vi "Documentation.vi"   [LabVIEW 2019, in "Inst.RP100.lvlib" / "Inst.RP100.lvclass"]
uses:
  Inst.RP100.lvclass
  7f3c9b6f-0033-4804-bc48-630b6ca02c12.vi
  7f3c9b6f-0033-4804-bc48-630b6ca02c12.vi/dae691d2-a16d-43f7-880e-3d4c6070a6ed.vi
  7f3c9b6f-0033-4804-bc48-630b6ca02c12.vi/01ba8764-a54b-435f-b6e6-8e2e51a5d755.vi
  <userlib>/LevyLab/Instrument Framework/Instrument/API/Instrument.sendMessageToProcess (string).vi
  <vilib>/Utility/Data Type/Get Type Information.vi
  <vilib>/JDP Science/JSONtext/JSON text to Variant.vi
  <userlib>/LevyLab/Instrument Framework/Instrument/Instrument.lvclass
  <vilib>/JKI/JKI SMO/SMO/SMO.lvclass
  Typedefs/Inst.RP100.Commands--Enum.ctl
  Typedefs/Inst.RP100.getAll--Cluster.ctl
  Typedefs/Inst.RP100.Configuration--Cluster.ctl
  Inst UI.RP100/Inst UI.RP100.lvclass
  Inst UI.RP100/Inst UI.RP100.UI--Cluster.ctl
  <vilib>/JKI/JKI SMO/SMO.UI/SMO.UI.lvclass
  <userlib>/LevyLab/Instrument Framework/Instrument UI/Instrument UI.lvclass
  <vilib>/JDP Science/JSONtext/LVClass Serializer/JSONtext LVClass Serializer.lvclass
  <userlib>/LevyLab/RemoteControl/RemoteControl/RemoteControl.lvclass
  C:/Program Files (x86)/National Instruments/LabVIEW 2019/user.lib/LevyLab/Instrument Framework/Instrument Types/Strain/Instrument.Strain.lvclass
  C:/Program Files (x86)/National Instruments/LabVIEW 2019/user.lib/LevyLab/Instrument Framework/Instrument/Instrument.lvclass
  C:/Program Files (x86)/National Instruments/LabVIEW 2019/vi.lib/JKI/JKI SMO/SMO/SMO.lvclass
  C:/Program Files (x86)/National Instruments/LabVIEW 2019/user.lib/LevyLab/Instrument Framework/Instrument UI/Instrument UI.lvclass
  C:/Program Files (x86)/National Instruments/LabVIEW 2019/vi.lib/JKI/JKI SMO/SMO.UI/SMO.UI.lvclass
types:
  T1 = typedef "Inst.RP100.lvlib/Inst.RP100.lvclass/Inst.RP100.getAll--Cluster.ctl" = cluster{"OutputStateCh1":string, "OutputStateCh2":string, "LevelCh1":dbl, "LevelCh2":dbl, "SlewCh1":dbl, "SlewCh2":dbl, "MeasuredVCh1":dbl, "MeasuredVCh2":dbl, "MeasuredICh1":dbl, "MeasuredICh2":dbl}
  T2 = typedef "Inst.RP100.lvlib/Inst.RP100.lvclass/Inst.RP100.Configuration--Cluster.ctl" = cluster{"Example Setting 1":dbl, "Example Setting 2":dbl, "Example Setting 3":string}
  T3 = typedef "Inst.RP100.lvlib/Inst.RP100.lvclass/Inst.RP100.Commands--Enum.ctl" = enum16{"setState", "setLevel", "getLevel"}
  T4 = typedef "Inst.RP100.lvlib/Inst UI.RP100.lvclass/Inst UI.RP100.UI--Cluster.ctl" = cluster{"Ch1 (V)":dbl, "Ch2 (V)":dbl, "Slew (V/s)":dbl}
  T5 = typedef "Instrument.lvlib/Instrument.lvclass/PublicEvents--Cluster.ctl" = cluster{"MessageFromProcess":refnum<user-event>}
  T6 = typedef "Instrument.lvlib/Instrument.lvclass/PrivateEvents--Cluster.ctl" = cluster{"MessageToProcess":refnum<user-event>, "LogData":refnum<user-event>}
  T7 = typedef "Inst.RP100.lvlib/Inst.RP100.lvclass/PublicEvents--Cluster.ctl" = cluster{"MessageFromProcess":refnum<user-event>}
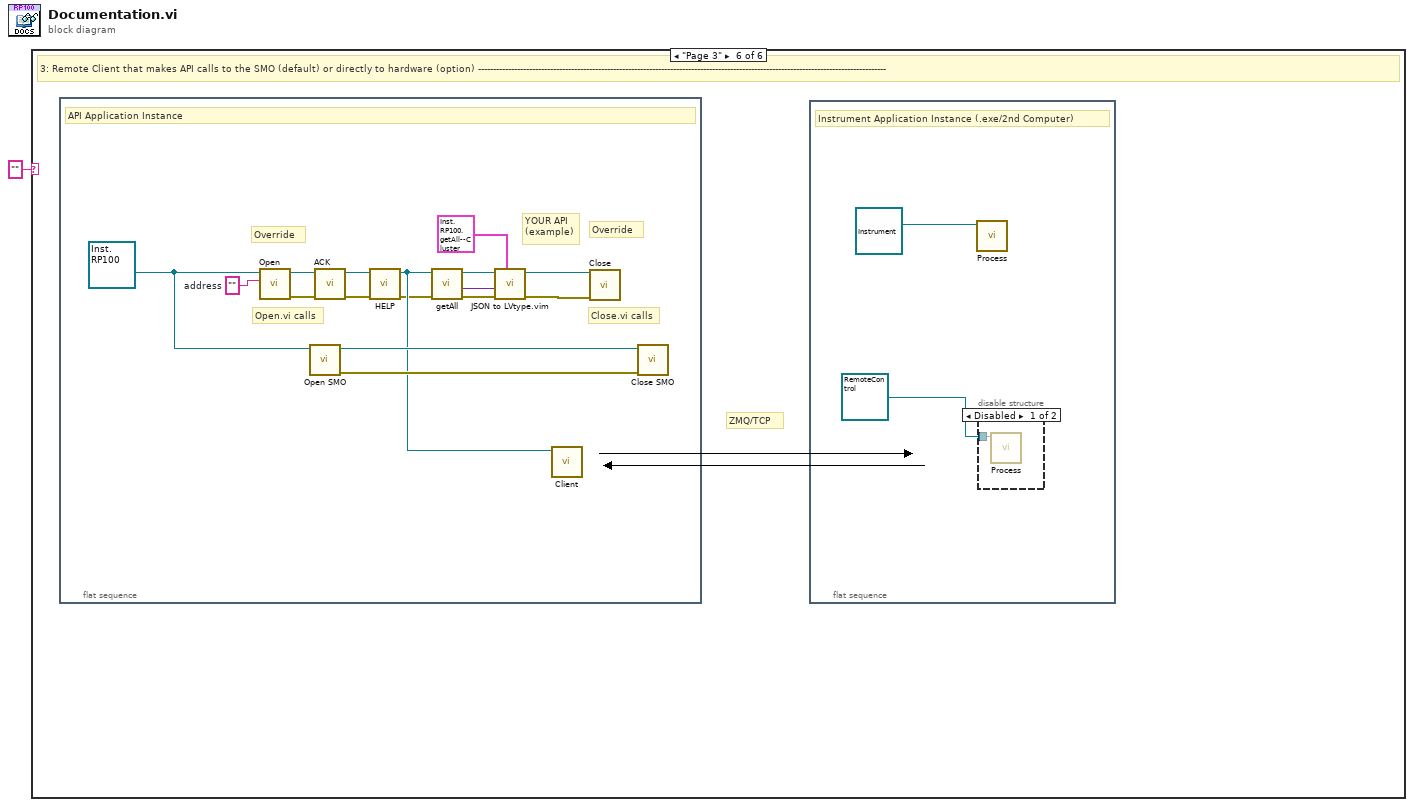
[diagram p0: block diagram]
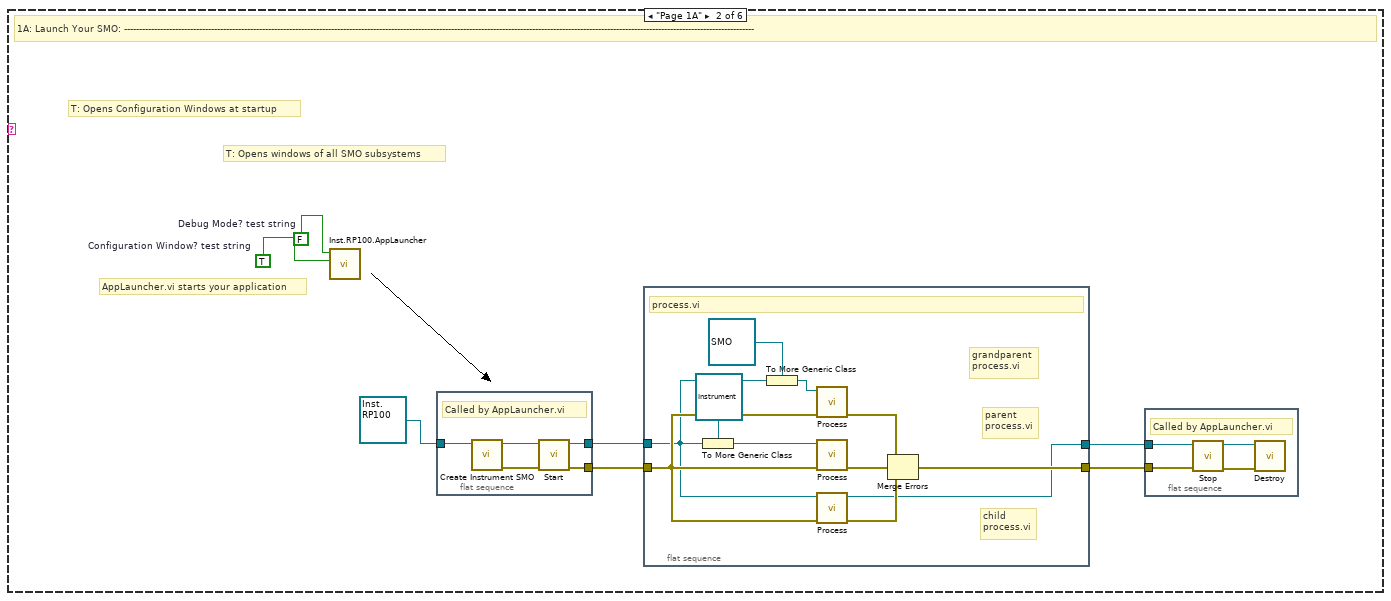
[diagram p3: hidden frame]
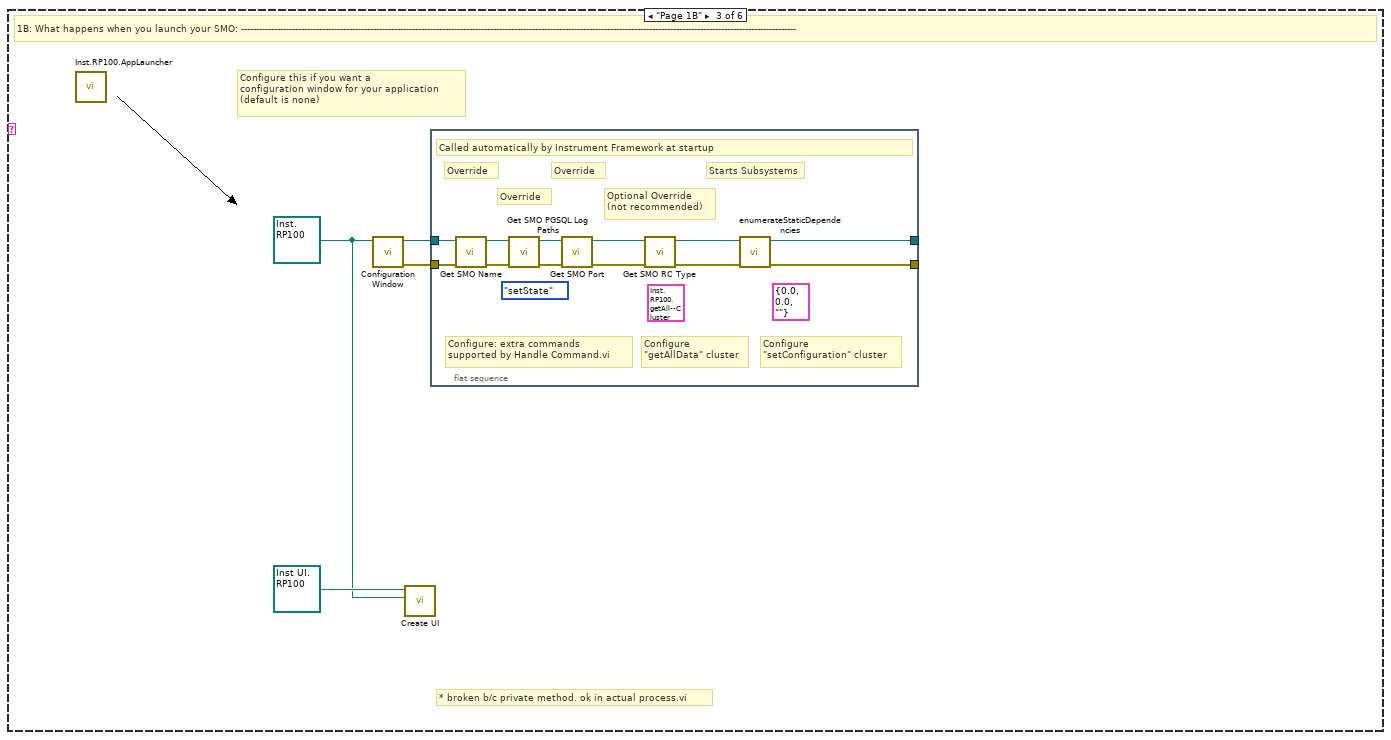
[diagram p4: hidden frame]
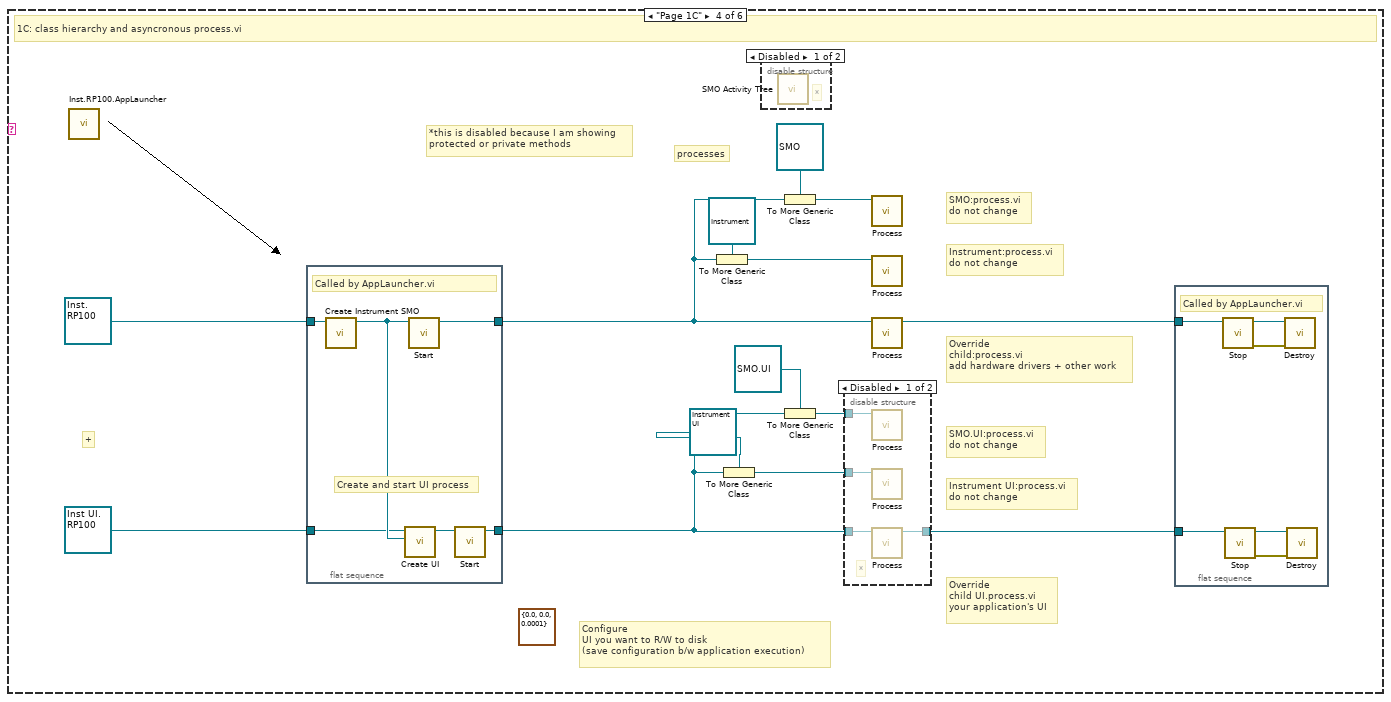
[diagram p5: hidden frame]
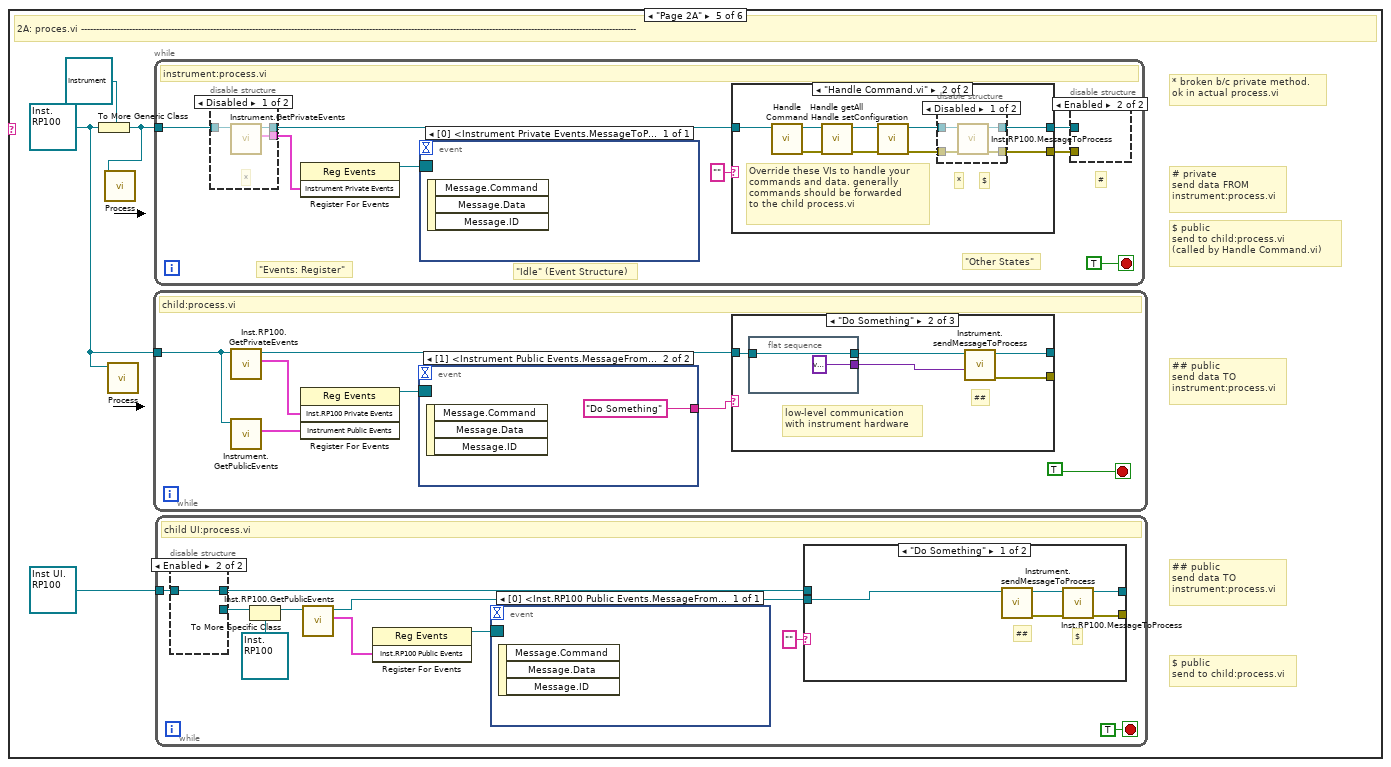
[diagram p8: hidden frame]
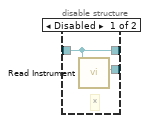
[diagram p10: hidden frame]
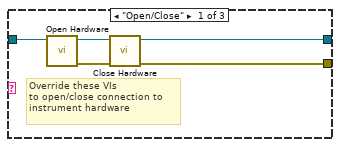
[diagram p11: hidden frame]
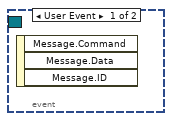
[diagram p13: hidden frame]
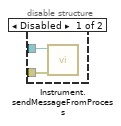
[diagram p14: hidden frame]
diagram:
  n1 = case shown="\"Page 3\"" "" {
    frame Default {
    }
    frame "Page 1A" {
      w7 = TRUE  # Configuration Window? test string
      w8 = FALSE  # Debug Mode? test string
      # "AppLauncher.vi starts your application"
      # "T: Opens windows of all SMO subsystems"
      # "T: Opens Configuration Windows at startup"
      # "1A: Launch Your SMO: ------------------------------------------------------------------------------------------------------------------------------------------------------------------------------------------------------------------"
      n2 = call "Inst.RP100.AppLauncher.vi"("Config Window"=w7, "Debug Mode"=w8) -> ()  [unwired: 9 in, 1 out]
      n3 = flat-sequence {
        tunnel: [w26] -> w3
        tunnel: [w25] -> w5
        tunnel: refnum<class "Inst.RP100.lvclass"> refnum ("Instrument.Template.lvclass") -> [w24]
        frame #0 {
          # "Called by AppLauncher.vi"
          n4 = call <userlib>:"Create Instrument SMO.vi"("Instrument in"=w24) -> ("error out"=w27:errorcluster, "Instrument out"=w28:refnum<class "Inst.RP100.lvclass">)  [unwired: 9 in]
          n5 = call <vilib>:"Start.vi"("error in (no error)"=w27, "SMO"=w28) -> ("error out"=w25:errorcluster, "SMO out"=w26:refnum<class "Inst.RP100.lvclass">)  [unwired: 8 in]
        }
      }
      n6 = flat-sequence {
        tunnel: [w19] -> w6
        tunnel: w5 -> [w17]
        tunnel: [w12] -> w4
        tunnel: w3 -> [w11]
        frame #0 {
          # "child\nprocess.vi"
          # "grandparent\nprocess.vi"
          # "parent\nprocess.vi"
          # "process.vi"
          n7 = To More Generic Class(target class=refnum<class "Instrument.lvclass"> refnum ("Instrument.lvlib:Instrument.lvclass"), reference=w11) -> (generic class reference=w16:refnum<class "Instrument.lvclass">)
          n8 = To More Generic Class(target class=refnum<class "SMO.lvclass"> refnum ("smo.lvlib:SMO.lvclass"), reference=w11) -> (generic class reference=w18:refnum<class "SMO.lvclass">)
          n9 = call-dynamic "Process.vi"("error in"=w17, "SMO"=w18) -> ("error out"=w13:errorcluster)  [unwired: 8 in, 1 out]
          n10 = call-dynamic "Process.vi"("error in"=w17, "Instrument"=w16) -> ("error out"=w15:errorcluster)  [unwired: 8 in, 1 out]
          n11 = call-dynamic "Process.vi"("error in"=w17, "Inst.RP100"=w11) -> ("error out"=w14:errorcluster, "Inst.RP100 out"=w12:refnum<class "Inst.RP100.lvclass">)  [unwired: 8 in]
          n12 = Merge Errors(w13, w15, w14) -> (w19:errorcluster)
        }
      }
      n13 = flat-sequence {
        tunnel: w4 -> [w21]
        tunnel: w6 -> [w20]
        frame #0 {
          # "Called by AppLauncher.vi"
          n14 = call <vilib>:"Stop.vi"("error in (no error)"=w20, "SMO"=w21) -> ("error out"=w23:errorcluster, "SMO out"=w22:refnum<class "Inst.RP100.lvclass">)  [unwired: 8 in]
          n15 = call <vilib>:"Destroy.vi"("error in (no error)"=w23, "SMO"=w22) -> ()  [unwired: 9 in, 1 out]
        }
      }
    }
    frame "Page 1B" {
      w29 = refnum<class "Inst.RP100.lvclass"> refnum ("Instrument.Template.lvclass")
      # "* broken b/c private method. ok in actual process.vi"
      # "Configure this if you want a\nconfiguration window for your application\n(default is none)"
      # "1B: What happens when you launch your SMO: -----------------------------------------------------------------------------------------------------------------------------------------------------------------------------------------"
      n16 = call "Inst.RP100.AppLauncher.vi"() -> ()  [unwired: 11 in, 1 out]
      n17 = call-dynamic "Configuration Window.vi"("Inst.RP100 in"=w29) -> ("error out"=w31:errorcluster, "Inst.RP100 out"=w32:refnum<class "Inst.RP100.lvclass">)  [unwired: 9 in]
      n18 = call <userlib>:"Create UI.vi"("Instrument in"=w29, "Instrument UI"=refnum<class "Inst UI.RP100.lvclass"> refnum ("Instrument UI.Template.lvclass")) -> ()  [unwired: 8 in, 2 out]
      n19 = flat-sequence {
        tunnel: w32 -> [w40]
        tunnel: w31 -> [w35]
        tunnel: [w34] -> _
        tunnel: [w33] -> _
        frame #0 {
          (unwired) T2 {"Example Setting 1"=0.0, "Example Setting 2"=0.0, "Example Setting 3"=""} ("Configuration")
          (unwired) T1 {"OutputStateCh1"="", "OutputStateCh2"="", "LevelCh1"=0.0, "LevelCh2"=0.0, "SlewCh1"=0.0, "SlewCh2"=0.0, "MeasuredVCh1"=0.0, "MeasuredVCh2"=0.0, "MeasuredICh1"=0.0, "MeasuredICh2"=0.0} ("getAll")
          (unwired) Inst.RP100.Commands--Enum."setState" ("Commands")
          # "Configure\n\"setConfiguration\" cluster"
          # "Configure\n\"getAllData\" cluster"
          # "Configure: extra commands\nsupported by Handle Command.vi"
          # "Starts Subsystems"
          # "Override"
          # "Override"
          # "Override"
          # "Optional Override\n(not recommended)"
          # "Called automatically by Instrument Framework at startup"
          n20 = call-dynamic "Get SMO Name.vi"("error in (no error)"=w35, "Inst.RP100 in"=w40) -> ("error out"=w38:errorcluster, "Inst.RP100 out"=w39:refnum<class "Inst.RP100.lvclass">)  [unwired: 7 in, 1 out]
          n21 = call-dynamic "Get SMO PGSQL Log Paths.vi"("error in (no error)"=w38, "Inst.RP100 in"=w39) -> ("error out"=w36:errorcluster, "Inst.RP100 out"=w37:refnum<class "Inst.RP100.lvclass">)  [unwired: 7 in, 1 out]
          n22 = call-dynamic "Get SMO Port.vi"("error in (no error)"=w36, "Inst.RP100Instrument in"=w37) -> ("error out"=w41:errorcluster, "Inst.RP100Instrument out"=w42:refnum<class "Inst.RP100.lvclass">)  [unwired: 7 in, 1 out]
          n23 = call-dynamic "Get SMO RC Type.vi"("error in (no error)"=w41, "Instrument in"=w42) -> ("error out"=w43:errorcluster, "Instrument out"=w44:refnum<class "Inst.RP100.lvclass">)  [unwired: 7 in, 1 out]
          n24 = call-dynamic "enumerateStaticDependencies.vi"("error in (no error)"=w43, "Instrument"=w44) -> ("error out"=w34:errorcluster, "Instrument out"=w33:refnum<class "Inst.RP100.lvclass">)  [unwired: 7 in, 1 out]
        }
      }
    }
    frame "Page 1C" {
      (unwired) T4 {"Ch1 (V)"=0.0, "Ch2 (V)"=0.0, "Slew (V/s)"=0.0001} ("UI")
      # "processes"
      # "SMO.UI:process.vi\ndo not change"
      # "Instrument UI:process.vi\ndo not change"
      # "Override\nchild:process.vi\nadd hardware drivers + other work"
      # "SMO:process.vi\ndo not change"
      # "Instrument:process.vi\ndo not change"
      # "*this is disabled because I am showing\nprotected or private methods"
      # "Configure\nUI you want to R/W to disk\n(save configuration b/w application execution)"
      # "Override\nchild UI.process.vi\nyour application's UI"
      # "+"
      # "1C: class hierarchy and asyncronous process.vi"
      n25 = call "Inst.RP100.AppLauncher.vi"() -> ()  [unwired: 11 in, 1 out]
      n26 = flat-sequence {
        tunnel: [w74] -> w57
        tunnel: refnum<class "Inst.RP100.lvclass"> refnum ("Instrument.Template.lvclass") -> [w73]
        tunnel: refnum<class "Inst UI.RP100.lvclass"> refnum ("Instrument UI.Template.lvclass") -> [w71]
        tunnel: [w69] -> w55
        frame #0 {
          # "Create and start UI process"
          # "Called by AppLauncher.vi"
          n27 = call <userlib>:"Create Instrument SMO.vi"("Instrument in"=w73) -> ("Instrument out"=w72:refnum<class "Inst.RP100.lvclass">)  [unwired: 9 in, 1 out]
          n28 = call <userlib>:"Create UI.vi"("Instrument in"=w72, "Instrument UI"=w71) -> ("Instrument UI out"=w70:refnum<class "Inst UI.RP100.lvclass">)  [unwired: 8 in, 1 out]
          n29 = call <vilib>:"Start.vi"("SMO"=w72) -> ("SMO out"=w74:refnum<class "Inst.RP100.lvclass">)  [unwired: 9 in, 1 out]
          n30 = call <vilib>:"Start.vi"("SMO"=w70) -> ("SMO out"=w69:refnum<class "Inst UI.RP100.lvclass">)  [unwired: 9 in, 1 out]
        }
      }
      n31 = To More Generic Class(target class=refnum<class "Instrument.lvclass"> refnum ("Instrument.lvlib:Instrument.lvclass"), reference=w57) -> (generic class reference=w52:refnum<class "Instrument.lvclass">)
      n32 = To More Generic Class(target class=refnum<class "Instrument UI.lvclass"> refnum ("Instrument.lvlib:Instrument UI.lvclass"), reference=w55) -> (generic class reference=w51:refnum<class "Instrument UI.lvclass">)
      n33 = disable-structure shown="Disabled" {
        frame Disabled {
          # "*"
          n34 = call <vilib>:"SMO Activity Tree.vi"() -> ()  [unwired: 12 in]
        }
        frame Enabled {
        }
      }
      n35 = To More Generic Class(target class=refnum<class "SMO.lvclass"> refnum ("smo.lvlib:SMO.lvclass"), reference=w57) -> (generic class reference=w53:refnum<class "SMO.lvclass">)
      n36 = To More Generic Class(target class=refnum<class "SMO.UI.lvclass"> refnum ("smo.lvlib:SMO.UI.lvclass"), reference=w55) -> (generic class reference=w50:refnum<class "SMO.UI.lvclass">)
      n37 = disable-structure shown="Disabled" {
        disable-tunnel: w55 -> [w62 _]
        disable-tunnel: [w61 _] -> w54
        disable-tunnel: w51 -> [w60 _]
        disable-tunnel: w50 -> [w59 _]
        frame Disabled {
          # "*"
          n38 = call-dynamic "Process.vi"("SMO.UI"=w59) -> ()  [unwired: 9 in, 2 out]
          n39 = call-dynamic "Process.vi"("Instrument UI in"=w60) -> ()  [unwired: 9 in, 2 out]
          n40 = call-dynamic "Process.vi"("Inst UI.RP100"=w62) -> ("Inst UI.RP100 out"=w61:refnum<class "Inst UI.RP100.lvclass">)  [unwired: 9 in, 1 out]
        }
        frame Enabled {
        }
      }
      n41 = call-dynamic "Process.vi"("SMO"=w53) -> ()  [unwired: 9 in, 2 out]
      n42 = call-dynamic "Process.vi"("Instrument"=w52) -> ()  [unwired: 9 in, 2 out]
      n43 = call-dynamic "Process.vi"("Inst.RP100"=w57) -> ("Inst.RP100 out"=w58:refnum<class "Inst.RP100.lvclass">)  [unwired: 9 in, 1 out]
      n44 = flat-sequence {
        tunnel: w58 -> [w66]
        tunnel: w54 -> [w64]
        frame #0 {
          # "Called by AppLauncher.vi"
          n45 = call <vilib>:"Stop.vi"("SMO"=w66) -> ("error out"=w68:errorcluster, "SMO out"=w67:refnum<class "Inst.RP100.lvclass">)  [unwired: 9 in]
          n46 = call <vilib>:"Stop.vi"("SMO"=w64) -> ("error out"=w65:errorcluster, "SMO out"=w63:refnum<class "Inst UI.RP100.lvclass">)  [unwired: 9 in]
          n47 = call <vilib>:"Destroy.vi"("error in (no error)"=w68, "SMO"=w67) -> ()  [unwired: 9 in, 1 out]
          n48 = call <vilib>:"Destroy.vi"("error in (no error)"=w65, "SMO"=w63) -> ()  [unwired: 9 in, 1 out]
        }
      }
    }
    frame "Page 2A" {
      w76 = refnum<class "Inst.RP100.lvclass"> refnum ("Instrument.Template.lvclass")
      # "## public\nsend data TO\ninstrument:process.vi"
      # "$ public\nsend to child:process.vi"
      # "## public\nsend data TO\ninstrument:process.vi"
      # "$ public\nsend to child:process.vi\n(called by Handle Command.vi)"
      # "# private\nsend data FROM\ninstrument:process.vi"
      # "* broken b/c private method.\nok in actual process.vi"
      # "2A: proces.vi -----------------------------------------------------------------------------------------------------------------------------------------------------------------------------------------"
      n49 = To More Generic Class(target class=refnum<class "Instrument.lvclass"> refnum ("Instrument.lvlib:Instrument.lvclass"), reference=w76) -> (generic class reference=w77:refnum<class "Instrument.lvclass">)
      n50 = call-dynamic "Process.vi"("Instrument"=w77) -> ()  [unwired: 9 in, 2 out]
      n51 = call-dynamic "Process.vi"("Inst.RP100"=w76) -> ()  [unwired: 9 in, 2 out]
      n52 = while {
        tunnel: w76 -> [w100]
        stop <- TRUE stop-if-true
        # "child:process.vi"
        n53 = call "Inst.RP100.GetPrivateEvents.vi"("Inst.RP100 in"=w100) -> ("Inst.RP100 Private Events"=w104:cluster{"MessageToProcess":refnum<user-event>}, "Inst.RP100 out"=w102:refnum<class "Inst.RP100.lvclass">)  [unwired: 8 in, 1 out]
        n54 = call <userlib>:"Instrument.GetPublicEvents.vi"("Instrument"=w100) -> ("Instrument Public Events"=w101:T5)  [unwired: 8 in, 2 out]
        n55 = register-events(w104, w101) -> (reference out=w103:refnum<event-registration>)  [unwired: 2 in, 1 out]
        n56 = event shown="[1] <Instrument Public Events.MessageFromProcess>: User Event" {
          selector: w103 -> [_ _]
          dyn-events: _ -> [_ _]
          timeout: _ -> [_ _]
          tunnel: [_ "Do Something"] -> w98
          event User Event {
            n57 = event-data() -> ()  [unwired: 1 in, 3 out]
          }
          event User Event {
            n58 = event-data() -> ()  [unwired: 1 in, 3 out]
          }
        }
        n59 = case shown="\"Do Something\"" w98 {
          tunnel: w102 -> [w107 w112 w117]
          tunnel: [w106 w114 w117] -> _
          tunnel: [w105 w113 _] -> _
          frame "Open/Close" {
            # "Override these VIs\nto open/close connection to\ninstrument hardware"
            n60 = call-dynamic "Open Hardware.vi"("Inst.RP100 in"=w107) -> ("error out"=w109:errorcluster, "Inst.RP100 out"=w108:refnum<class "Inst.RP100.lvclass">)  [unwired: 9 in]
            n61 = call-dynamic "Close Hardware.vi"("error in (no error)"=w109, "Inst.RP100 in"=w108) -> ("error out"=w105:errorcluster, "Inst.RP100 out"=w106:refnum<class "Inst.RP100.lvclass">)  [unwired: 8 in]
          }
          frame "Do Something" {
            # "##"
            # "low-level communication\nwith instrument hardware"
            n62 = flat-sequence {
              tunnel: w112 -> [w116]
              tunnel: [w116] -> w111
              tunnel: [variant ("Data")] -> w110
              frame #0 {
              }
            }
            n63 = call-poly <userlib>:"Instrument.sendMessageToProcess.vi"("Data"=w110, "Instrument"=w111) -> ("error out"=w113:errorcluster, "Instrument out"=w114:refnum<class "Inst.RP100.lvclass">)  [unwired: 8 in]
          }
          frame Default {
          }
        }
      }
      n64 = while {
        tunnel: w77 -> [w125]
        stop <- TRUE stop-if-true
        # "#"
        # "\"Other States\""
        # "\"Idle\" (Event Structure)"
        # "\"Events: Register\""
        # "instrument:process.vi"
        n65 = disable-structure shown="Disabled" {
          disable-tunnel: w125 -> [w147 w148]
          disable-tunnel: [w146 w148] -> w124
          disable-tunnel: [w145 _] -> w123
          frame Disabled {
            # "*"
            n66 = call <userlib>:"Instrument.GetPrivateEvents.vi"("Instrument"=w147) -> ("Instrument Private Events"=w145:T6, "Instrument out"=w146:refnum<class "Instrument.lvclass">)  [unwired: 8 in, 1 out]
          }
          frame Enabled {
          }
        }
        n67 = register-events(w123) -> (reference out=w122:refnum<event-registration>)  [unwired: 2 in, 1 out]
        n68 = event shown="[0] <Instrument Private Events.MessageToProcess>: User Event" {
          selector: w122 -> [_]
          dyn-events: _ -> [_]
          timeout: _ -> [_]
          event User Event {
            n69 = event-data() -> ()  [unwired: 1 in, 3 out]
          }
        }
        n70 = case shown="\"Handle Command.vi\"" "" {
          tunnel: w124 -> [w129 w138]
          tunnel: [w129 w132] -> w121
          tunnel: [_ w131] -> w120
          frame Default {
          }
          frame "Handle Command.vi" {
            # "*"
            # "$"
            # "Override these VIs to handle your\ncommands and data. generally \ncommands should be forwarded\nto the child process.vi"
            n71 = call-dynamic "Handle Command.vi"("Instrument in"=w138) -> ("error out"=w134:errorcluster, "Instrument out"=w137:refnum<class "Instrument.lvclass">)  [unwired: 7 in, 2 out]
            n72 = call-dynamic "Handle getAll.vi"("error in (no error)"=w134, "Instrument in"=w137) -> ("error out"=w135:errorcluster, "Instrument out"=w136:refnum<class "Instrument.lvclass">)  [unwired: 7 in, 1 out]
            n73 = call-dynamic "Handle setConfiguration.vi"("error in (no error)"=w135, "Instrument in"=w136) -> ("error out"=w130:errorcluster, "Instrument out"=w133:refnum<class "Instrument.lvclass">)  [unwired: 8 in]
            n74 = disable-structure shown="Disabled" {
              disable-tunnel: w133 -> [w139 w144]
              disable-tunnel: [w142 w144] -> w132
              disable-tunnel: [w141 w143] -> w131
              disable-tunnel: w130 -> [w140 w143]
              frame Disabled {
                n75 = call "Inst.RP100.MessageToProcess.vi"("error in (no error)"=w140, "Inst.RP100 in"=w139) -> ("error out"=w141:errorcluster, "Inst.RP100 out"=w142:refnum<class "Inst.RP100.lvclass">)  [unwired: 8 in]
              }
              frame Enabled {
              }
            }
          }
        }
        n76 = disable-structure shown="Enabled" {
          disable-tunnel: w121 -> [w127 _]
          disable-tunnel: w120 -> [w128 _]
          frame Disabled {
            n77 = call <userlib>:"Instrument.sendMessageFromProcess.vi"("error in (no error)"=w128, "Instrument"=w127) -> ()  [unwired: 8 in, 2 out]
          }
          frame Enabled {
          }
        }
      }
      n78 = while {
        tunnel: refnum<class "Inst UI.RP100.lvclass"> refnum ("Instrument UI.Template.lvclass") -> [w87]
        stop <- TRUE stop-if-true
        # "child UI:process.vi"
        n79 = disable-structure shown="Enabled" {
          disable-tunnel: w87 -> [w95 w97]
          disable-tunnel: [w96 _] -> w85
          disable-tunnel: [w95 w97] -> w81
          frame Disabled {
            # "*"
            n80 = call <userlib>:"Read Instrument.vi"("Instrument UI in"=w95) -> ("Instrument"=w96:refnum<class "Instrument.lvclass">)  [unwired: 8 in, 2 out]
          }
          frame Enabled {
          }
        }
        n81 = To More Specific Class(target class=refnum<class "Inst.RP100.lvclass"> refnum ("Instrument.Template.lvclass"), reference=w85) -> (specific class reference=w84:refnum<class "Inst.RP100.lvclass">)  [unwired: 1 in, 1 out]
        n82 = call "Inst.RP100.GetPublicEvents.vi"("Inst.RP100 in"=w84) -> ("Inst.RP100 Public Events"=w82:T7, "Inst.RP100 out"=w80:refnum<class "Inst.RP100.lvclass">)  [unwired: 8 in, 1 out]
        n83 = register-events(w82) -> (reference out=w83:refnum<event-registration>)  [unwired: 2 in, 1 out]
        n84 = event shown="[0] <Inst.RP100 Public Events.MessageFromProcess>: User Event" {
          selector: w83 -> [_]
          dyn-events: _ -> [_]
          timeout: _ -> [_]
          event User Event {
            n85 = event-data() -> ()  [unwired: 1 in, 3 out]
          }
        }
        n86 = case shown="\"Do Something\"" "" {
          tunnel: w81 -> [_ _]
          tunnel: [w93 w94] -> _
          tunnel: [w92 _] -> _
          tunnel: w80 -> [w90 w94]
          frame "Do Something" {
            # "##"
            # "$"
            n87 = call-poly <userlib>:"Instrument.sendMessageToProcess.vi"("Instrument"=w90) -> ("error out"=w91:errorcluster, "Instrument out"=w89:refnum<class "Inst.RP100.lvclass">)  [unwired: 9 in]
            n88 = call "Inst.RP100.MessageToProcess.vi"("error in (no error)"=w91, "Inst.RP100 in"=w89) -> ("error out"=w92:errorcluster, "Inst.RP100 out"=w93:refnum<class "Inst.RP100.lvclass">)  [unwired: 8 in]
          }
          frame Default {
          }
        }
      }
    }
    frame "Page 3" {
      # "ZMQ/TCP"
      # "3: Remote Client that makes API calls to the SMO (default) or directly to hardware (option) ----------------------------------------------------------------------------------------------------------------------------------------"
      n89 = flat-sequence {
        frame #0 {
          w161 = ""  # address
          w166 = refnum<class "Inst.RP100.lvclass"> refnum ("Instrument.Template.lvclass")
          # "Close.vi calls"
          # "Open.vi calls"
          # "YOUR API\n(example)"
          # "Override"
          # "Override"
          # "API Application Instance"
          n90 = call-dynamic "Open.vi"("address"=w161, "Inst.RP100 in"=w166) -> ("error out"=w165:errorcluster, "Inst.RP100 out"=w164:refnum<class "Inst.RP100.lvclass">)  [unwired: 8 in]
          n91 = call <userlib>:"Open SMO.vi"("Instrument in"=w166) -> ("error out"=w159:errorcluster, "Instrument out"=w160:refnum<class "Inst.RP100.lvclass">)  [unwired: 9 in]
          n92 = call <userlib>:"ACK.vi"("error in (no error)"=w165, "Instrument in"=w164) -> ("error out"=w163:errorcluster, "Instrument out"=w162:refnum<class "Inst.RP100.lvclass">)  [unwired: 7 in, 1 out]
          n93 = call <userlib>:"HELP.vi"("error in (no error)"=w163, "Instrument in"=w162) -> ("error out"=w156:errorcluster, "Instrument in"=w157:refnum<class "Inst.RP100.lvclass">)  [unwired: 7 in, 1 out]
          n94 = call <userlib>:"getAll.vi"("error in (no error)"=w156, "Instrument in"=w157) -> ("error out"=w153:errorcluster, "getAll"=w154:variant, "Instrument out"=w158:refnum<class "Inst.RP100.lvclass">)  [unwired: 7 in]
          n95 = call "JSON to LVtype.vim"("type"=T1 {"OutputStateCh1"="", "OutputStateCh2"="", "LevelCh1"=0.0, "LevelCh2"=0.0, "SlewCh1"=0.0, "SlewCh2"=0.0, "MeasuredVCh1"=0.0, "MeasuredVCh2"=0.0, "MeasuredICh1"=0.0, "MeasuredICh2"=0.0} ("getAll"), "error in (no error)"=w153, "JSON Data in"=w154) -> ("error out"=w152:errorcluster)  [unwired: 7 in, 1 out]
          n96 = call-dynamic "Client.vi"("Instrument in"=w157) -> ()  [unwired: 7 in, 4 out]
          n97 = call-dynamic "Close.vi"("error in (no error)"=w152, "Inst.RP100 in"=w158) -> ()  [unwired: 8 in, 2 out]
          n98 = call <userlib>:"Close SMO.vi"("error in (no error)"=w159, "Instrument in"=w160) -> ()  [unwired: 8 in, 2 out]
        }
      }
      n99 = flat-sequence {
        frame #0 {
          # "Instrument Application Instance (.exe/2nd Computer)"
          n100 = call-dynamic "Process.vi"("Instrument"=refnum<class "Instrument.lvclass"> refnum ("Instrument.lvlib:Instrument.lvclass")) -> ()  [unwired: 9 in, 2 out]
          n101 = disable-structure shown="Disabled" {
            disable-tunnel: refnum<class "RemoteControl.lvclass"> refnum ("RemoteControl.lvlib:RemoteControl.lvclass") -> [w151 _]
            frame Disabled {
              n102 = call-dynamic "Process.vi"("RemoteControl"=w151) -> ()  [unwired: 9 in, 2 out]
            }
            frame Enabled {
            }
          }
        }
      }
    }
  }
